vi "Verify User PIN.vi"(8 "error in (no error)":errorcluster, 11 "PIN":string) -> (0 "error out":errorcluster, 1 "Account Balance":dbl, 2 "ATM Message":string, 3 "Verified?":bool, 4 "User PIN":string, 5 "Account Holder":string)   [LabVIEW 2025]
doc: "Verifies User from the Accounts.csv file. It can also be used to gather the account balance."
uses:
  <vilib>/Utility/file.llb/Read Delimited Spreadsheet (string).vi
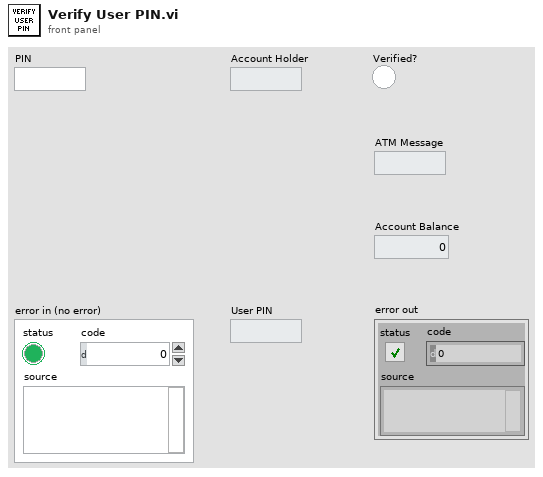
[diagram p1: front panel]
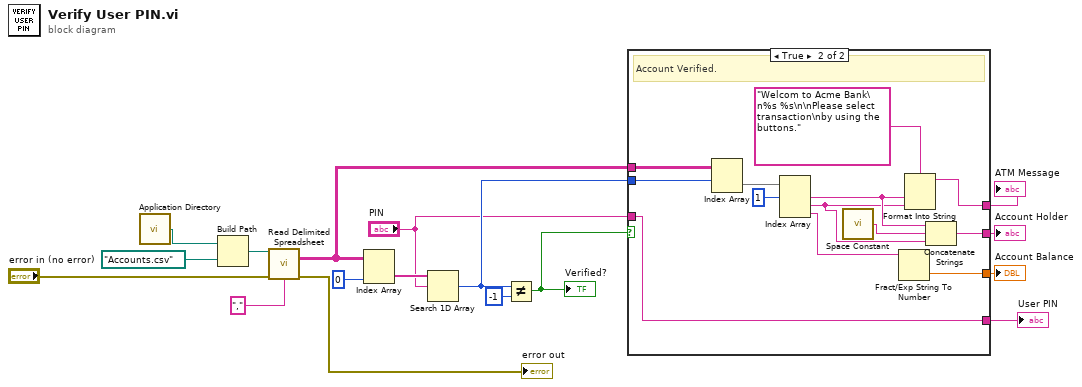
[diagram p0: block diagram]
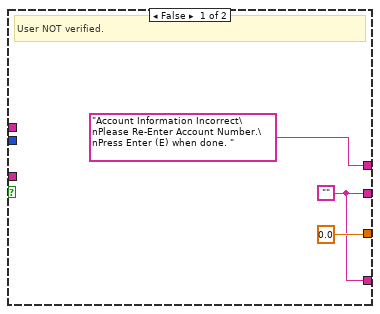
[diagram p2: hidden frame]
diagram:
  n1 = call <vilib>:"Application Directory.vi"() -> ("Application Directory"=w13:path)
  n2 = Build Path(base path=w13, name or relative path=path "Accounts.csv" ("file path (dialog if empty)")) -> (appended path=w16:path)
  n3 = call-poly <vilib>:"Read Delimited Spreadsheet.vi"("file path (dialog if empty)"=w16, "error in (no error)"="error in (no error)", "delimiter (\\t)"="," ("delimiter (\\t)")) -> ("all rows"=w7:string[][], "error out"=→"error out":errorcluster)  [unwired: 7 in, 4 out]
  n4 = Index Array(array=w7, index (col)=0) -> (element=w11:string[])  [unwired: 1 in]
  n5 = Search 1D Array(1D array=w11, element="PIN") -> (index of element=w6:i32)  [unwired: 1 in]
  n6 = Not Equal?(x=w6, y=-1) -> (x != y?=w8:bool)
  "Verified?" <- w8
  n7 = case shown="True" w8 {
    tunnel: w7 -> [_ w33]
    tunnel: w6 -> [_ w32]
    tunnel: ["Account Information Incorrect\nPlease Re-Enter Account Number.\nPress Enter (E) when done. " w28] -> w5
    tunnel: [0.0 w26] -> w4
    tunnel: [w18 w22] -> w3
    tunnel: "PIN" -> [_ w21]
    tunnel: [w18 w21] -> w1
    frame False {
      w18 = "" ("Empty String Constant")
      # "User NOT verified."
    }
    frame True {
      # "Account Verified."
      n8 = Index Array(array=w33, index (row)=w32) -> (element=w31:string[])  [unwired: 1 in]
      n9 = Index Array(array=w31, index #1=1 ("index")) -> (element #1=w25:string, element #2=w24:string, element #3=w27:string)  [unwired: 2 in]
      n10 = call <vilib>:"Space Constant.vi"() -> ("String"=w23:string)
      n11 = Fract/Exp String To Number(string=w27) -> (number=w26:dbl)  [unwired: 3 in, 1 out]
      n12 = Format Into String(format string="Welcom to Acme Bank\n%s %s\n\nPlease select transaction\nby using the buttons.", w25, w24) -> (resulting string=w28:string)  [unwired: 2 in, 1 out]
      n13 = Concatenate Strings(w25, w23, w24) -> (w22:string)
    }
  }
  "ATM Message" <- w5
  "Account Balance" <- w4
  "Account Holder" <- w3
  "User PIN" <- w1
